vi "Get Executable Attributes.vi"(8 "error in (no error)":errorcluster, 11 "ReadCommand in":refnum<class "ReadCommand.lvclass">) -> (0 "error out":errorcluster, 2 "Executable Attributes":T1, 3 "ReadCommand out":refnum<class "ReadCommand.lvclass">)   [LabVIEW 2023, in "HAF.lvlib" / "ReadCommand.lvclass"]
doc: "Provides a set of attributes that are used to control how the Driver should run the Executable on an Instrument."
uses:
  ReadCommand.lvclass
  ReadCommand.lvclass/ReadCommand.ctl
  WriteCommand/WriteCommand.lvclass
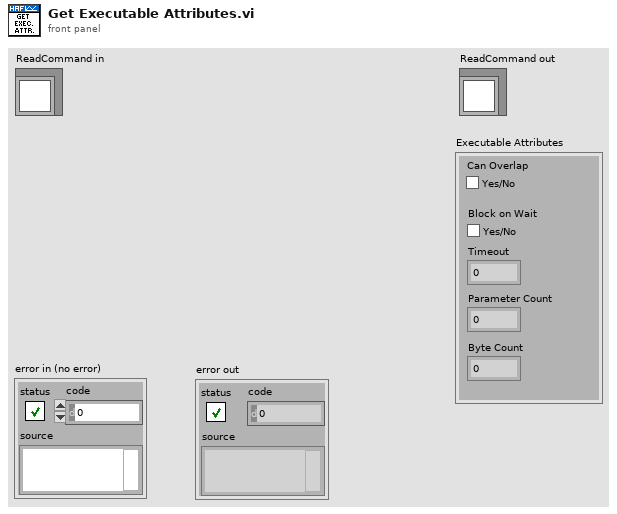
[diagram p1: front panel]
types:
  T1 = cluster{"Can Overlap":bool, "Block on Wait":bool, "Timeout":u32, "Byte Count":u32, "Parameter Count":u32}
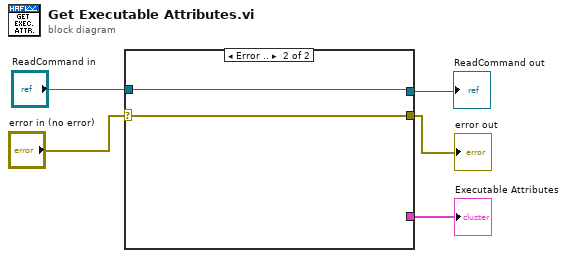
[diagram p0: block diagram]
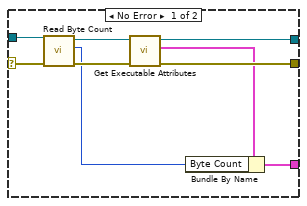
[diagram p2: hidden frame]
diagram:
  n1 = case shown="Error .." "error in (no error)" {
    selector: "error in (no error)" -> [w10 w15]
    tunnel: "ReadCommand in" -> [w11 w16]
    tunnel: [w14 w16] -> w3
    tunnel: [w13 w15] -> w2
    tunnel: [w6 _] -> w1
    frame No Error {
      n2 = call-dynamic "Read Byte Count.vi"("error in (no error)"=w10, "ReadCommand in"=w11) -> ("error out"=w8:errorcluster, "Byte Count"=w7:u32, "ReadCommand out"=w9:refnum<class "ReadCommand.lvclass">)  [unwired: 7 in]
      n3 = call-parent "Get Executable Attributes.vi"("error in (no error)"=w8, "WriteCommand in"=w9) -> ("error out"=w13:errorcluster, "Executable Attributes"=w12:T1, "WriteCommand out"=w14:refnum<class "ReadCommand.lvclass">)  [unwired: 7 in]
      n4 = Bundle By Name(cluster=w12, "Byte Count"=w7) -> (w6:T1)
    }
    frame Error {
    }
  }
  "error out" <- w2
  "ReadCommand out" <- w3
  "Executable Attributes" <- w1
